vi "S7Com_WRT+READ(SubVI).vi"(4 "Write_Data":T6, 5 "error in":errorcluster, 6 "timeout ms (25000)":i32, 7 "RW_CMD":T1={"Read Length"=1, "Data Block #"=1, "S7_Add_Area"=132, "Start Address"=0, "S7_Transport_Size"=2, "S7_Function"=4} {"S7_Function" items=["Read"=4, "Write"=5]; "S7_Transport_Size" items=["BIT"=1, "BYTE"=2, "CHAR"=3, "WORD"=4, "INT"=5, "DWORD"=6, "DINT"=7, "REAL"=8]; "S7_Add_Area" items=["P Area"=128, "I Area"=129, "O Area"=130, "M Area"=131, "DB Area"=132, "Counter"=40, "Timer"=41]}, 8 "connection ID in":refnum<k5>) -> (0 "error out":errorcluster, 1 "Error":bool, 2 "Read_Data":T6, 3 "connection ID out":refnum<k5>)   [LabVIEW 2019]
doc: "Holds the subVIs used in a S7 Protocol Request/Respone transaction."
uses:
  S7Com_Data_Array.ctl
  S7Com_RW_CMD.ctl
  S7Com_Address_Area.ctl
  S7Com_Start_Add.ctl
  S7Com_Transport_Size.ctl
  S7Com_Function.ctl
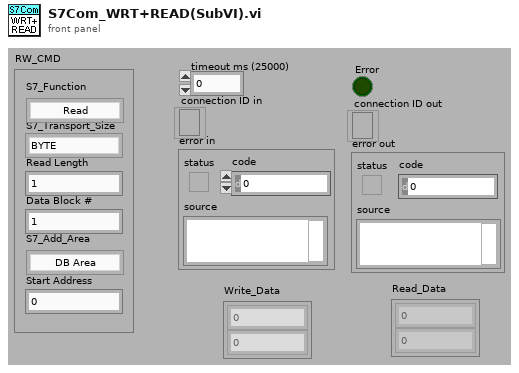
[diagram p1: front panel]
types:
  T1 = typedef "S7Com_RW_CMD.ctl" = cluster{"Read Length":u16, "Data Block #":u16, "S7_Add_Area":T2, "Start Address":T3, "S7_Transport_Size":T4, "S7_Function":T5}
  T2 = typedef "S7Com_Address_Area.ctl" = u8
  T3 = typedef "S7Com_Start_Add.ctl" = u16
  T4 = typedef "S7Com_Transport_Size.ctl" = u8
  T5 = typedef "S7Com_Function.ctl" = u8
  T6 = typedef "S7Com_Data_Array.ctl" = i32[]
  T7 = typedef "S7Com_HexByteArray.ctl" = T8[]
  T8 = typedef "S7Com_HexByte.ctl" = u8
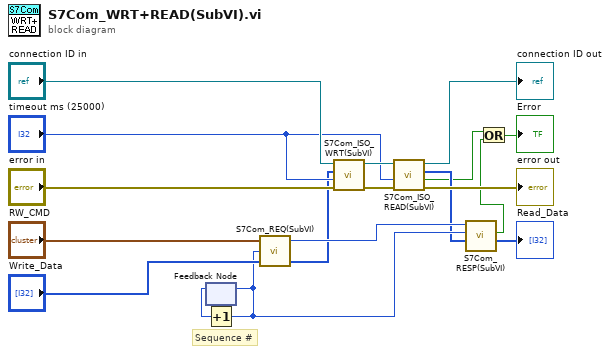
[diagram p0: block diagram]
diagram:
  # "Sequence #"
  n1 = feedback #1() -> (w10:u16)  [unwired: 1 out]
  n2 = Increment(x=w10) -> (x+1=w7:u16)
  n3 = feedback-in #1(w7) -> ()
  n4 = call "S7Com_REQ(SubVI).vi"("Write Data"="Write_Data", "Sequence#"=w7, "RW_CMD"="RW_CMD") -> ("Out Data"=w5:T7, "S7_Transport_Size"=w6:T4)  [unwired: 1 out]
  n5 = call "S7Com_ISO_WRT(SubVI).vi"("error in"="error in", "timeout ms (25000)"="timeout ms (25000)", "TPDU_In"=w5, "connection ID in"="connection ID in") -> ("error out"=w13:errorcluster, "connection ID out"=w14:refnum<k5>)  [unwired: 2 out]
  n6 = call "S7Com_ISO_READ(SubVI).vi"("error in"=w13, "timeout ms (25000)"="timeout ms (25000)", "connection ID in"=w14) -> ("error out"=→"error out":errorcluster, "Error"=w2:bool, "TPDU Data"=w4:T7, "connection ID out"=→"connection ID out":refnum<k5>)  [unwired: 1 out]
  n7 = call "S7Com_RESP(SubVI).vi"("PDU_In"=w4, "Seq# In"=w7, "Transport Size In"=w6) -> ("Output_Data"=→"Read_Data":T6, "Error"=w1:bool)  [unwired: 7 out]
  n8 = Or(x=w2, y=w1) -> (x .or. y?=→"Error":bool)
